vi "KDH_4th_Ex3Challenge3_1-24-17.vi"() -> ()   [LabVIEW 2014, in "Harris_MacMaster_4th_LEGORobotics_11-29-16.lvrbt"]
uses:
  Harris_MacMaster_4th_LEGORobotics_11-29-16.lvrbt
  <vilib>/NXT/Dual Mode Library/Sensors/EV3_Ultrasonic_CM.vi
panel:
  out "Error?":bool
  in  "Stop Button":bool
  out "Distance LED":bool
  out "Wall Proximity":string
  in  "Min Distance":dbl
  in  "Max Distance":dbl
  out "Current Distance":dbl
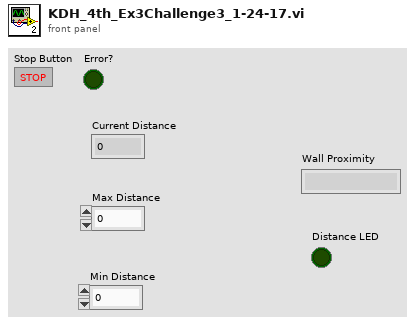
[diagram p1: front panel]
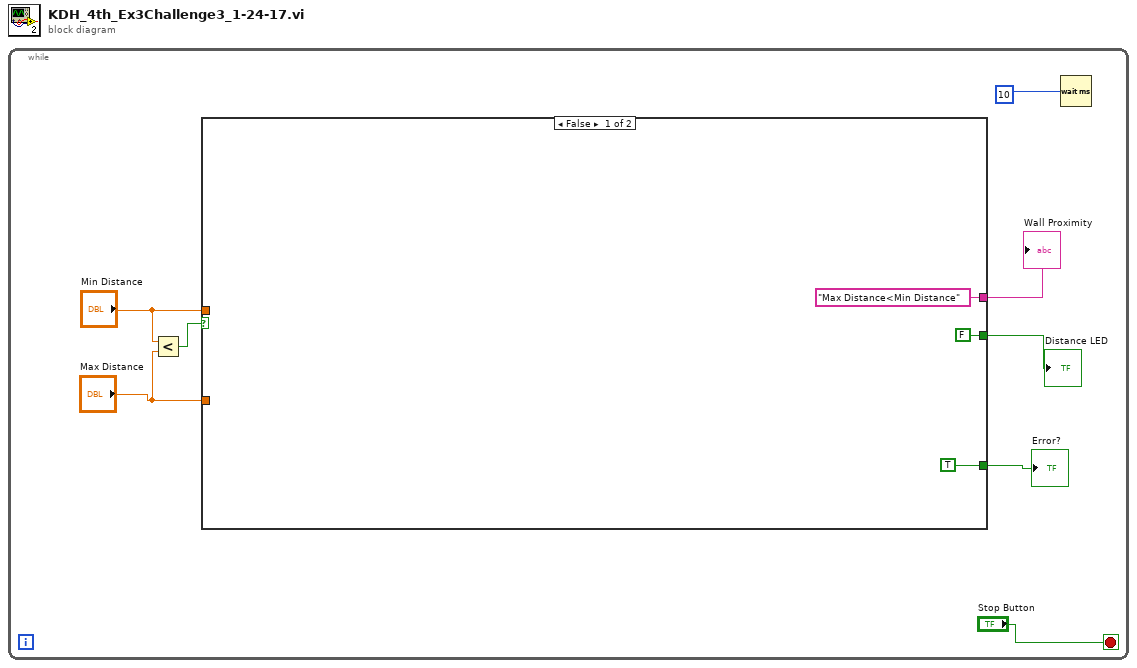
[diagram p0: block diagram]
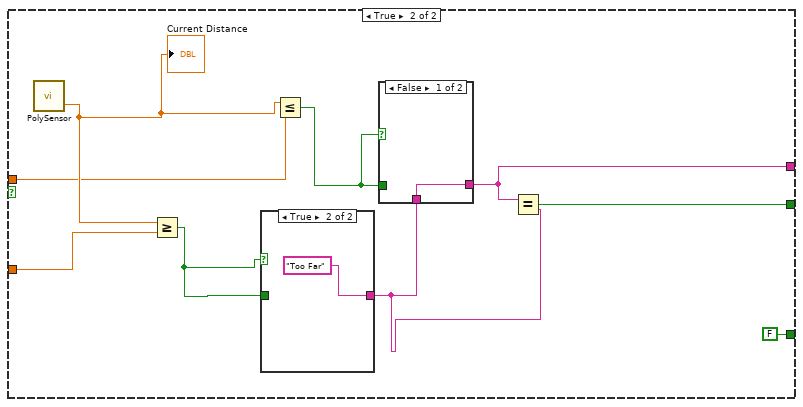
[diagram p2: hidden frame]
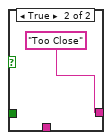
[diagram p3: hidden frame]
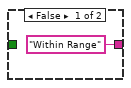
[diagram p4: hidden frame]
diagram:
  n1 = while {
    stop <- "Stop Button" stop-if-true
    n2 = Less?(x="Min Distance", y="Max Distance") -> (x < y?=w6:bool)
    n3 = case shown="False" w6 {
      tunnel: "Max Distance" -> [_ w19]
      tunnel: "Min Distance" -> [_ w18]
      tunnel: ["Max Distance<Min Distance" w17] -> w3
      tunnel: [FALSE w16] -> w2
      tunnel: [TRUE ("Error?") FALSE ("Error?")] -> w1
      frame False {
      }
      frame True {
        n4 = call-poly <vilib>:"PolySensor.vi"() -> ("Centimeters"=w20:sgl)  [unwired: 3 in, 1 out]
        "Current Distance" <- w20
        n5 = Greater Or Equal?(x=w20, y=w19) -> (x >= y?=w13:bool)
        n6 = case shown="True" w13 {
          tunnel: w13 -> [_ _]
          tunnel: ["Within Range" "Too Far"] -> w14
          frame False {
          }
          frame True {
          }
        }
        n7 = Less Or Equal?(x=w20, y=w18) -> (x <= y?=w12:bool)
        n8 = case shown="False" w12 {
          tunnel: w12 -> [_ _]
          tunnel: [w21 "Too Close"] -> w17
          tunnel: w14 -> [w21 _]
          frame False {
          }
          frame True {
          }
        }
        n9 = Equal?(x=w17, y=w14) -> (x = y?=w16:bool)
      }
    }
    "Wall Proximity" <- w3
    "Distance LED" <- w2
    "Error?" <- w1
    n10 = Wait (ms)(milliseconds to wait=u32 10 ("millisecond timer value")) -> ()  [unwired: 1 out]
  }
